vi "Flow 2016.vi"(5 "Descriptions":string[](array[string]), 6 "Array in":refnum<k24>[](array[refnum]), 8 "Flow Slope":dbl=37.99800109863281 format="%.2f", 9 "Offset":dbl format="%.1f") -> (2 "Sensor Cluster":T1, 3 "Flow (ml/min)":dbl format="%.2f", 4 "Array out":refnum<k24>[](array[refnum]))   [LabVIEW 2016]
uses:
  C:/Cascade-lv16-64/builds/Waterloo Main Program/cascade/data/ULx_LV.dll
  builds/Waterloo Main Program/cascade/data/ULx_LV.dll
  controls/MCC DAQ Readings.ctl
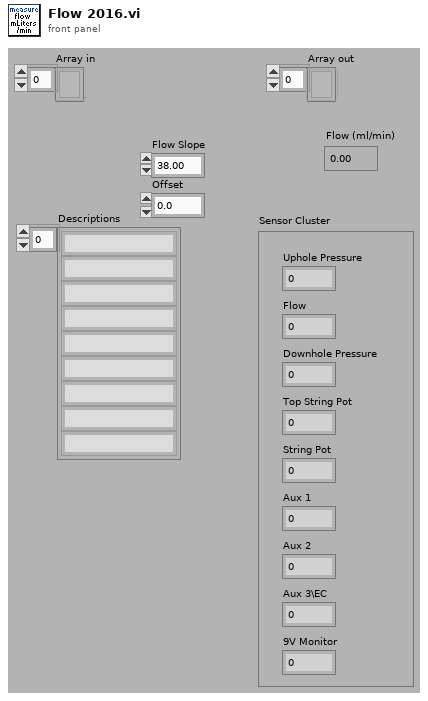
[diagram p1: front panel]
types:
  T1 = typedef "MCC DAQ Readings.ctl" = cluster{"Uphole Pressure":dbl, "Flow":dbl, "Downhole Pressure":dbl, "Top String Pot":dbl, "String Pot":dbl, "Aux 1":dbl, "Aux 2":dbl, "Aux 3\\EC":dbl, "9V Monitor":dbl}
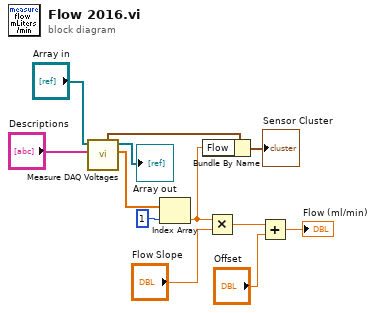
[diagram p0: block diagram]
diagram:
  n1 = call "Measure DAQ Voltages.vi"("Descriptions"="Descriptions", "Array in"="Array in") -> ("Raw Voltages"=w8:dbl[], "Array out"=→"Array out":refnum<k24>[], "Sensor Cluster"=w4:T1)  [unwired: 6 in, 1 out]
  n2 = Index Array(array=w8, index=1) -> (element=w2:dbl)
  n3 = Bundle By Name(cluster=w4, "Flow"=w2) -> (→"Sensor Cluster":T1)
  n4 = Multiply(x=w2, y="Flow Slope") -> (x*y=w12:dbl)
  n5 = Add(x=w12, y="Offset") -> (x+y=→"Flow (ml/min)":dbl)
